vi "LM Buffer.vi"(1 "FG Action (Read)":T2, 2 "LM Buffer In":T1(array[cluster])) -> (0 "LM Buffer Out":T1(array[cluster]))   [LabVIEW 2009]
uses:
  cRIO/Functional Global Variables/Actions for FG's.ctl
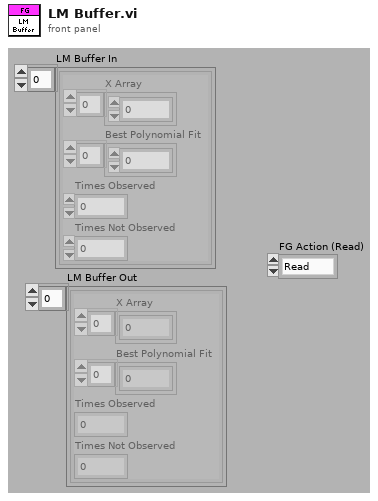
[diagram p1: front panel]
types:
  T1 = cluster{"X Array":dbl[], "Best Polynomial Fit":dbl[], "Times Observed":dbl, "Times Not Observed":dbl}[]
  T2 = typedef "Actions for FG's.ctl" = enum16{"Read", "Write"}
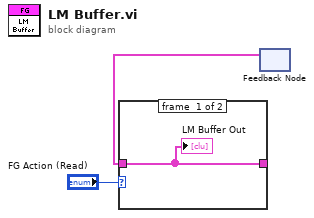
[diagram p0: block diagram]
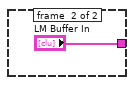
[diagram p2: hidden frame]
diagram:
  n1 = feedback #1() -> (w1:T1)  [unwired: 1 in]
  n2 = case shown="\"Read\", Default" "FG Action (Read)" {
    tunnel: [w4 "LM Buffer In"] -> w2
    tunnel: w1 -> [w4 _]
    frame #0 {
      "LM Buffer Out" <- w4
    }
    frame #1 {
    }
  }
